vi "Tree Control - Symbols.vi"() -> ()   [LabVIEW 2015, in "Utility.lvlib"]
uses:
  Utility.lvlib
panel:
  in  "Listbox":i32(listbox)
  # "The listbox shows the number assigned to the default symbols.\n\nThis can be used to set a treecontrol symbol."
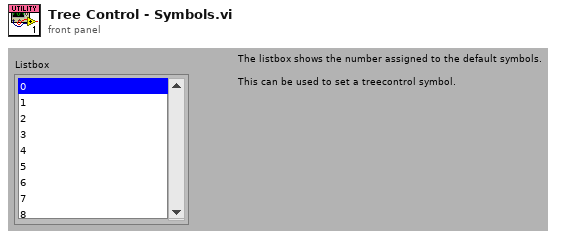
[diagram p1: front panel]
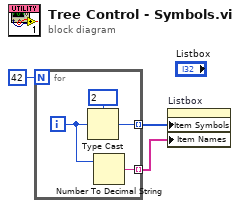
[diagram p0: block diagram]
diagram:
  n1 = for {
    N: 42 -> [_]
    tunnel: [w6] -> w2 mode=indexing
    tunnel: [w4] -> w1 mode=indexing
    i -> [w5]
    n2 = Type Cast(type=2, x=w5) -> (*(type *) &x=w6:i32)
    n3 = Number To Decimal String(number=w5) -> (decimal integer string=w4:string)  [unwired: 1 out]
  }
  n4 = property on="Listbox" class="LstBox (strict)"("Item Symbols"=w2, "Item Names"=w1) -> ()  [unwired: 2 in, 2 out]
